vi "Read 128 File.vi"(8 "错误输入":errorcluster, 11 "Path":path=path "E:/LCU6331 test/Procedure2/RFID_m645_Prodtest_LCU6331.128") -> (0 "错误输出":errorcluster, 1 "输出数组":string[](array[string]), 2 "line size":i32, 3 "path":path)   [LabVIEW 2009]
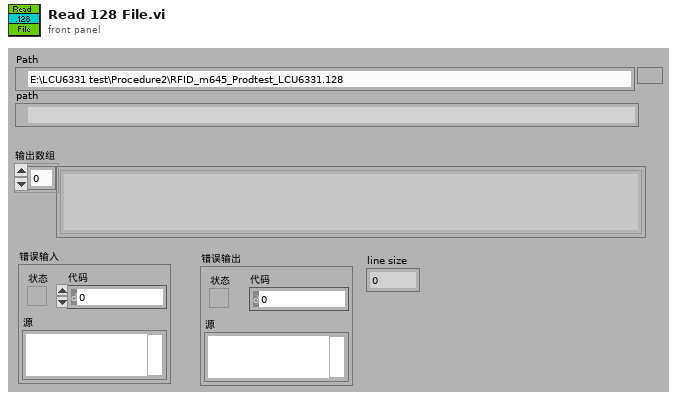
[diagram p1: front panel]
types:
  T1 = enum16{"open", "replace", "create", "open or create", "replace or create", "replace or create with confirmation"}
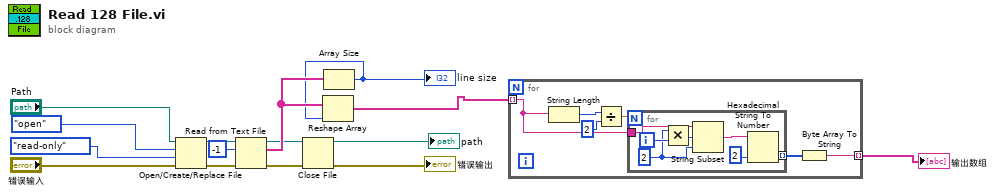
[diagram p0: block diagram]
diagram:
  n1 = Open/Create/Replace File(file path (use dialog)="Path", error in="错误输入", operation (0:open)=T1."open" ("操作(0:open)"), access (0:read/write)=enum16{"read/write", "read-only", "write-only"}."read-only" ("权限(0:read/write)")) -> (refnum out=w11:refnum<file>, error out=w12:errorcluster)  [unwired: 3 out]
  n2 = Read from Text File(file (use dialog)=w11, count=-1 ("计数"), error in=w12) -> (refnum out=w8:refnum<file>, text=w10:string[], error out=w7:errorcluster)  [unwired: 2 out]
  n3 = Close File(refnum=w8, error in=w7) -> (path=→"path":path, error out=→"错误输出":errorcluster)
  n4 = Array Size(array=w10) -> (size(s)=w5:i32)
  "line size" <- w5
  n5 = Reshape Array(w10, w5) -> (w2:string[])
  n6 = for {
    tunnel: w2 -> [w18] mode=indexing
    tunnel: [w16] -> w1 mode=indexing
    n7 = String Length(string=w18) -> (length=w21:i32)
    n8 = Divide(x=w21, y=2) -> (x/y=w19:dbl)
    n9 = for {
      N: w19 -> [_]
      tunnel: w18 -> [w28]
      tunnel: [w23] -> w17 mode=indexing
      i -> [w27]
      w26 = 2 ("length (rest)")
      n10 = Multiply(x=w26, y=w27) -> (x*y=w25:i32)
      n11 = String Subset(string=w28, offset (0)=w25, length (rest)=w26) -> (substring=w24:string)
      n12 = Hexadecimal String To Number(string=w24, default (0uL)=u8 2) -> (number=w23:u8)  [unwired: 2 out]
    }
    n13 = Byte Array To String(unsigned byte array=w17) -> (string=w16:string)
  }
  "输出数组" <- w1
